vi "SetOutput.vi"(3 "State":bool, 4 "error in":errorcluster, 5 "connection ID":refnum<k5>) -> (1 "error out":errorcluster, 2 "connection ID out":refnum<k5>)   [LabVIEW 2013]
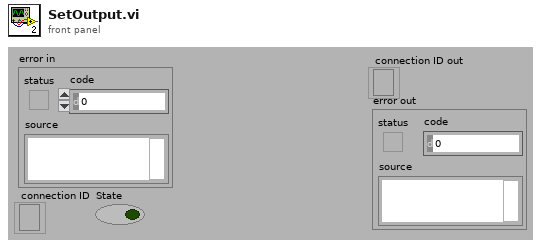
[diagram p1: front panel]
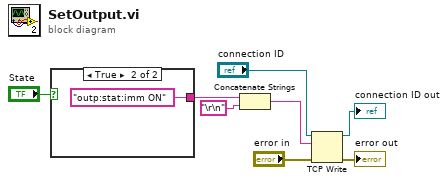
[diagram p0: block diagram]
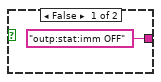
[diagram p2: hidden frame]
diagram:
  n1 = case shown="True" "State" {
    tunnel: ["outp:stat:imm OFF" ("data in") "outp:stat:imm ON" ("data in")] -> w2
    frame False {
    }
    frame True {
    }
  }
  n2 = Concatenate Strings(w2, "\r\n") -> (w3:string)
  n3 = TCP Write(connection ID="connection ID", data in=w3, error in (no error)="error in") -> (connection ID out=→"connection ID out":refnum<k5>, error out=→"error out":errorcluster)  [unwired: 2 out]
